vi "Inform.vi"(8 "error in (no error)":errorcluster, 10 "Message in":refnum<class "InformMessage.lvclass">, 11 "ImagingModeSPIM in":refnum<class "ImagingModeSPIM.lvclass">) -> (0 "error out":errorcluster, 3 "ImagingModeSPIM out":refnum<class "ImagingModeSPIM.lvclass">)   [LabVIEW 2012, in "ImagingModeSPIM.lvclass"]
doc: "The inform method processes the command inform'. \n\nThe command inform' is used for obtaining the latest instance data of the class. It also handles the current state of the observee and sets the 'ready' flag for the observee."
uses:
  ImagingModeSPIM.lvclass
  <vilib>/Distrio/Murmex/InformMessage/InformMessage.lvclass
  <vilib>/Distrio/Murmex/Murmex/Murmex.lvclass
  <vilib>/Distrio/Murmex/GenericMessage/GenericMessage.lvclass
  <vilib>/Distrio/Murmex/Message/Message.lvclass
panel:
  # "This method is called when the INFORM\ntrigger is sent. \n\nOverride this method when your component needs to\nrespond to this trigger. \n\nCall parent for proper implementation"
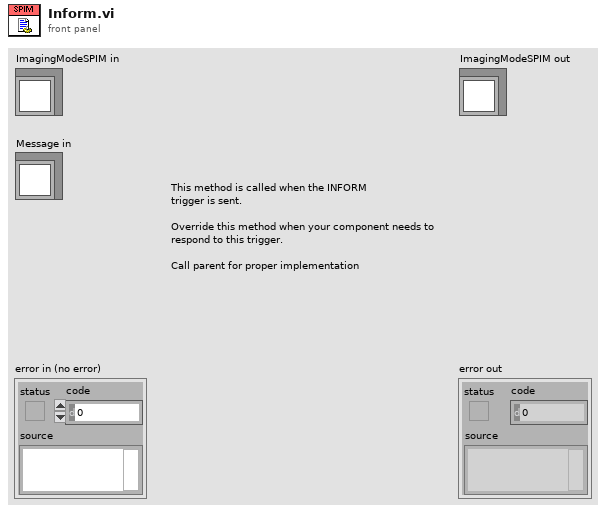
[diagram p1: front panel]
types:
  T1 = typedef "Murmex.lvlib/Murmex.lvclass/command_enum.ctl" = enum16{"null", "initialise", "reset", "terminate", "acknowledge", "update", "inspect", "inform", "proceed", "start", "stop", "fetch", "configure", "generic"}
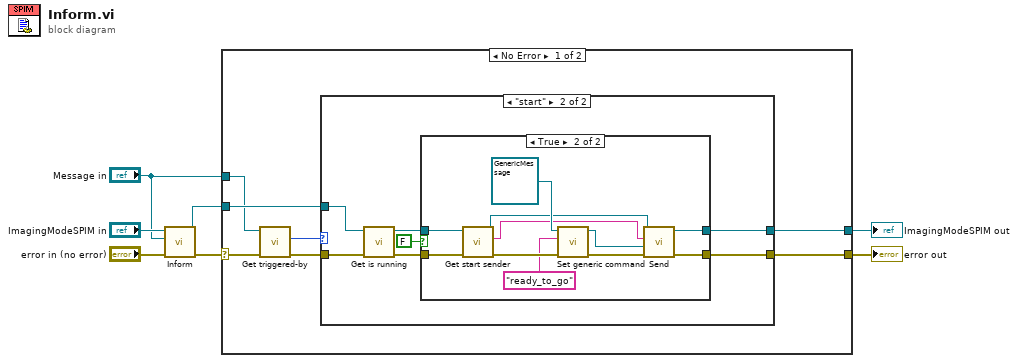
[diagram p0: block diagram]
diagram:
  n1 = call-parent "Inform.vi"("error in (no error)"="error in (no error)", "Message in"="Message in", "Murmex in"="ImagingModeSPIM in") -> ("error out"=w5:errorcluster, "Murmex out"=w4:refnum<class "ImagingModeSPIM.lvclass">)  [unwired: 7 in]
  n2 = case shown="No Error" w5 {
    selector: w5 -> [w11 w37]
    tunnel: w4 -> [w14 w38]
    tunnel: [w13 w38] -> w3
    tunnel: [w12 w37] -> w2
    tunnel: "Message in" -> [w9 _]
    frame No Error {
      n3 = call <vilib>:"Get triggered-by.vi"("error in (no error)"=w11, "Message in"=w9) -> ("error out"=w10:errorcluster, "triggered-by"=w8:T1)  [unwired: 7 in, 1 out]
      n4 = case shown="\"start\"" w8 {
        tunnel: w14 -> [w16 w23]
        tunnel: w10 -> [w15 w22]
        tunnel: [w16 w21] -> w13
        tunnel: [w15 w19] -> w12
        frame "null", Default {
        }
        frame "start" {
          n5 = call-dynamic "Get is running.vi"("error in (no error)"=w22, "ImagingModeSPIM in"=w23) -> ("error out"=w18:errorcluster, "ImagingModeSPIM out"=w20:refnum<class "ImagingModeSPIM.lvclass">)  [unwired: 7 in, 1 out]
          n6 = case shown="True" FALSE {
            tunnel: [w25 w29] -> w21
            tunnel: w20 -> [w25 w35]
            tunnel: [w24 w31] -> w19
            tunnel: w18 -> [w24 w36]
            frame False {
            }
            frame True {
              n7 = call-dynamic "Get start sender.vi"("error in (no error)"=w36, "ImagingModeSPIM in"=w35) -> ("error out"=w33:errorcluster, "start sender"=w27:string, "ImagingModeSPIM out"=w30:refnum<class "ImagingModeSPIM.lvclass">)  [unwired: 7 in]
              n8 = call <vilib>:"Set generic command.vi"("error in (no error)"=w33, "generic command"="ready_to_go", "GenericMessage in"=refnum<class "GenericMessage.lvclass"> refnum ("Message in")) -> ("error out"=w32:errorcluster, "GenericMessage out"=w28:refnum<class "GenericMessage.lvclass">)  [unwired: 7 in]
              n9 = call <vilib>:"Send.vi"("error in (no error)"=w32, "Message"=w28, "recipient"=w27, "Murmex in"=w30) -> ("error out"=w31:errorcluster, "Murmex out"=w29:refnum<class "ImagingModeSPIM.lvclass">)  [unwired: 6 in]
            }
          }
        }
      }
    }
    frame Error {
    }
  }
  "error out" <- w2
  "ImagingModeSPIM out" <- w3
